vi "Drive_Test_PIDs.vi"() -> ()   [LabVIEW 2019]
panel:
  in  "STOP":bool
  in  "initialAngle (degrees)":dbl
  in  "deltaGoal (degrees)":dbl=90.0
  out "goal angle":dbl=190.0
  in  "deltaP":dbl=0.0001
  in  "End P":dbl=0.001
  in  "Initial P":dbl=0.0001
  out "P":dbl=0.0010000000000000002
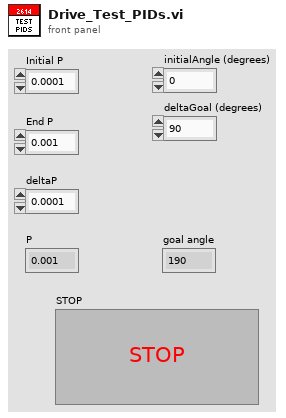
[diagram p1: front panel]
types:
  T1 = cluster{"Kp":dbl, "Ki":dbl, "Kd":dbl, "N-Diff":i32, "N-Int":i32, "Int Error Window":dbl, "Max Ouput":dbl, "Min Output":dbl}
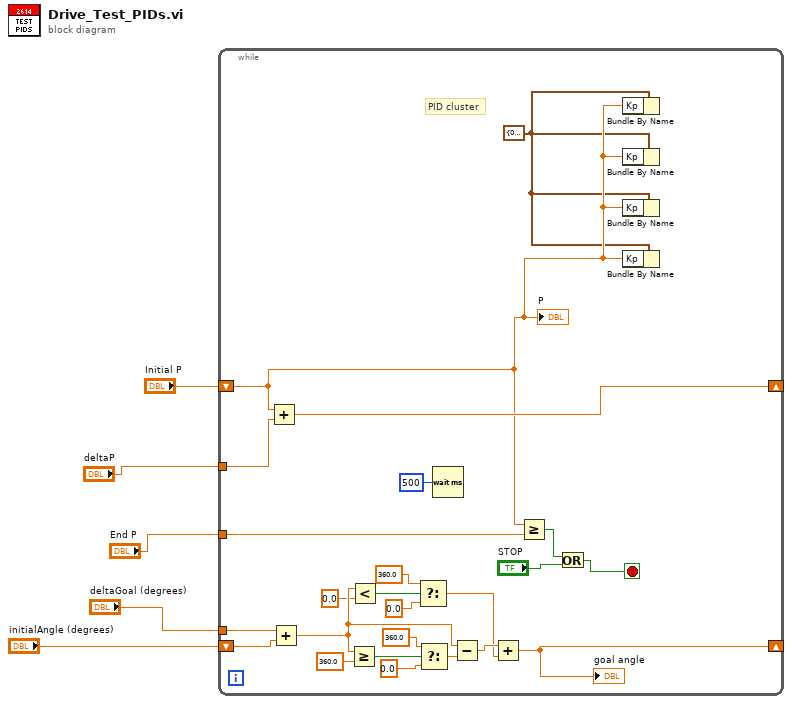
[diagram p0: block diagram]
diagram:
  n1 = while {
    shift-right: [w25] -> _
    shift-left: "Initial P" -> [w7]
    tunnel: "deltaP" -> [w29]
    tunnel: "End P" -> [w28]
    shift-right: [w10] -> _
    shift-left: "initialAngle (degrees)" -> [w24]
    tunnel: "deltaGoal (degrees)" -> [w23]
    stop <- w9 stop-if-true
    w6 = T1 {"Kp"=0.0, "Ki"=0.0, "Kd"=0.0, "N-Diff"=10, "N-Int"=10, "Int Error Window"=20.0, "Max Ouput"=0.5, "Min Output"=-0.5} ("Front_Left_PID")
    # "PID cluster"
    n2 = Add(x=w7, y=w29) -> (x+y=w25:dbl)
    n3 = Add(x=w23, y=w24) -> (x+y=w18:dbl)
    n4 = Greater Or Equal?(x=w18, y=360.0) -> (x >= y?=w21:bool)
    n5 = Less?(x=w18, y=0.0) -> (x < y?=w15:bool)
    n6 = Select(t=360.0, s=w15, f=0.0) -> (s? t:f=w11:dbl)
    n7 = Select(t=360.0, s=w21, f=0.0) -> (s? t:f=w19:dbl)
    n8 = Wait (ms)(milliseconds to wait=u32 500) -> ()  [unwired: 1 out]
    n9 = Subtract(x=w18, y=w19) -> (x-y=w12:dbl)
    n10 = Add(x=w12, y=w11) -> (x+y=w10:dbl)
    "goal angle" <- w10
    n11 = Greater Or Equal?(x=w7, y=w28) -> (x >= y?=w27:bool)
    n12 = Or(x=w27, y="STOP") -> (x .or. y?=w9:bool)
    n13 = Bundle By Name(cluster=w6, "Kp"=w7) -> ()  [unwired: 1 out]
    n14 = Bundle By Name(cluster=w6, "Kp"=w7) -> ()  [unwired: 1 out]
    n15 = Bundle By Name(cluster=w6, "Kp"=w7) -> ()  [unwired: 1 out]
    n16 = Bundle By Name(cluster=w6, "Kp"=w7) -> ()  [unwired: 1 out]
    "P" <- w7
  }
